vi "Axis_Jump Point.vi"(10 "Offset":T1, 11 "RobotPoints in":string[](array[string])) -> (0 "error out":errorcluster)   [LabVIEW 2019]
uses:
  LLB/Commonly VI/FilterPointNameToFloat.vi
panel:
  in  "error in (no error)":errorcluster
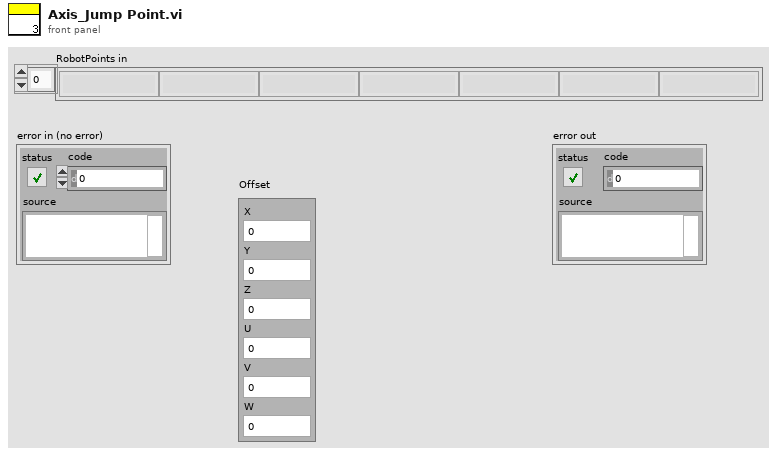
[diagram p1: front panel]
types:
  T1 = cluster{"X":dbl, "Y":dbl, "Z":dbl, "U":dbl, "V":dbl, "W":dbl}
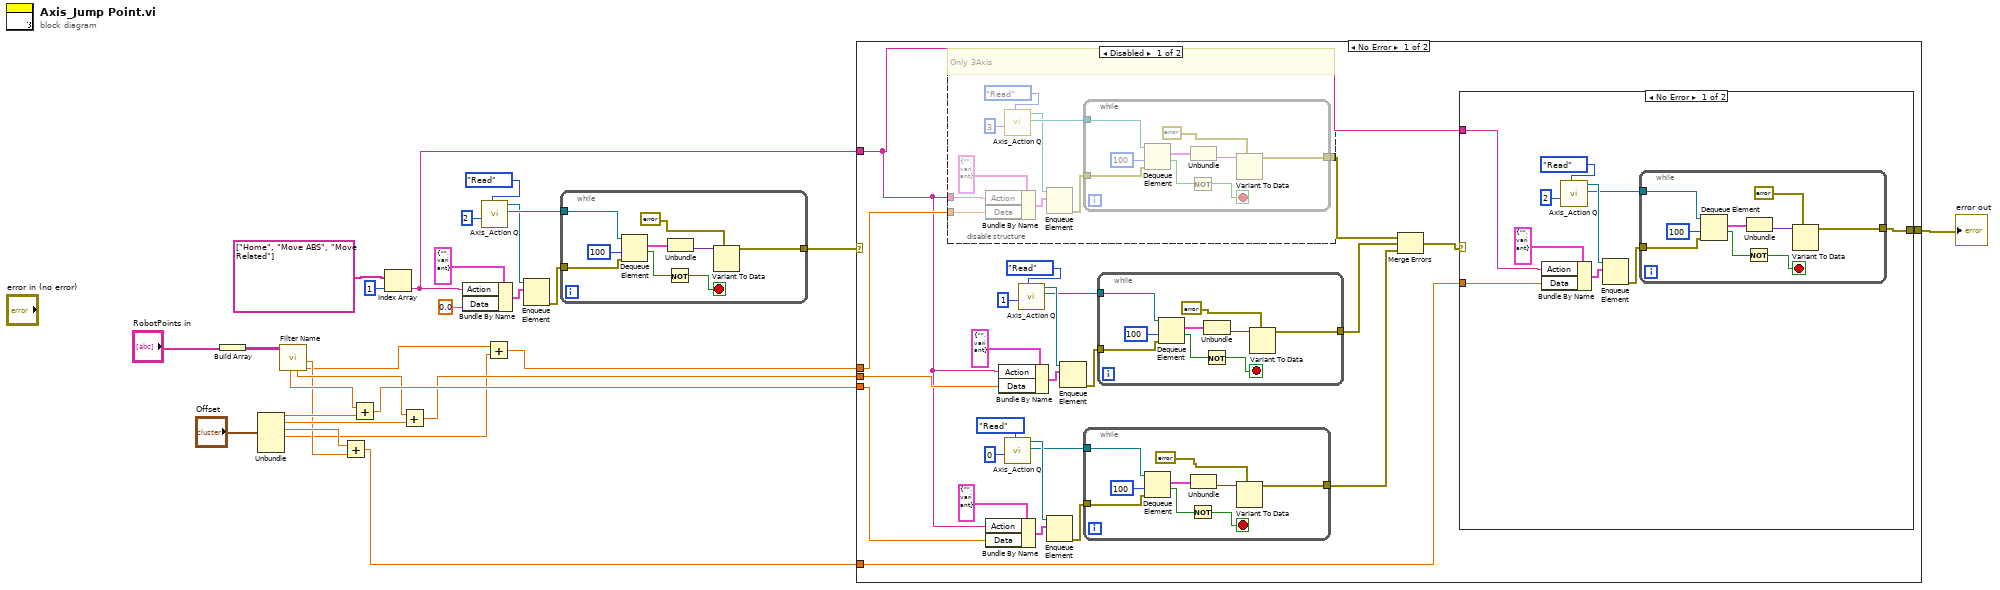
[diagram p0: block diagram]
diagram:
  n1 = Build Array("RobotPoints in") -> (w17:string[][])
  n2 = Unbundle("Offset") -> ("X"=w13:dbl, "Y"=w10:dbl, "Z"=w7:dbl, "U"=w3:dbl)  [unwired: 2 out]
  n3 = call-poly "Filter Name.vi"("RobotPoints in"=w17) -> ("U"=w2:dbl, "Z"=w6:dbl, "Y"=w9:dbl, "X"=w12:dbl)  [unwired: 4 in, 3 out]
  n4 = Add(x=w7, y=w6) -> (x+y=w5:dbl)
  n5 = Add(x=w12, y=w13) -> (x+y=w11:dbl)
  n6 = Index Array(array=string[] ["Home", "Move ABS", "Move Related"], index=1) -> (element=w18:string)
  n7 = Add(x=w9, y=w10) -> (x+y=w8:dbl)
  n8 = Bundle By Name(cluster=cluster{"Action":string, "Data":variant} {"Action"="", "Data"=variant} ("element"), "Action"=w18, "Data"=0.0) -> (w26:cluster{"Action":string, "Data":variant})
  n9 = call "Axis_Action Q.vi"("Enum"=enum16{"Initial", "Write", "Read"}."Read", "Axis Index"=2) -> ("Axis ActFeedBackQ Out"=w27:refnum<queue>, "Axis ActQ Out"=w25:refnum<queue>)  [unwired: 7 in, 1 out]
  n10 = Add(x=w2, y=w3) -> (x+y=w4:dbl)
  n11 = Enqueue Element(queue=w25, element=w26) -> (error out=w28:errorcluster)  [unwired: 2 in, 2 out]
  n12 = while {
    tunnel: w27 -> [w37]
    tunnel: w28 -> [w36]
    tunnel: [w29] -> w19
    stop <- w32 stop-if-true
    n13 = Dequeue Element(queue=w37, timeout in ms (-1)=100, error in (no error)=w36) -> (element=w34:cluster{"Action":string, "Data":variant}, timed out?=w33:bool)  [unwired: 2 out]
    n14 = Not(x=w33) -> (.not. x?=w32:bool)
    n15 = Unbundle(w34) -> ("Data"=w31:variant)  [unwired: 1 out]
    n16 = Variant To Data(type=errorcluster {"status"=FALSE, "code"=0, "source"=""} ("error constant"), Variant=w31) -> (data=w29:errorcluster)  [unwired: 1 in, 1 out]
  }
  n17 = case shown="No Error" w19 {
    selector: w19 -> [_ w119]
    tunnel: w18 -> [w40 _]
    tunnel: w11 -> [w47 _]
    tunnel: w8 -> [w46 _]
    tunnel: w4 -> [w45 _]
    tunnel: w5 -> [w39 _]
    tunnel: [w38 w119] -> w15
    frame No Error {
      n18 = disable-structure shown="Disabled" {
        disable-tunnel: w45 -> [w64 _]
        disable-tunnel: [w63 _] -> w44
        disable-tunnel: w40 -> [w62 _]
        frame Disabled {
          # "Only 3Axis"
          n19 = Bundle By Name(cluster=cluster{"Action":string, "Data":variant} {"Action"="", "Data"=variant} ("element"), "Action"=w62, "Data"=w64) -> (w69:cluster{"Action":string, "Data":variant})
          n20 = call "Axis_Action Q.vi"("Enum"=enum16{"Initial", "Write", "Read"}."Read", "Axis Index"=3) -> ("Axis ActFeedBackQ Out"=w70:refnum<queue>, "Axis ActQ Out"=w68:refnum<queue>)  [unwired: 7 in, 1 out]
          n21 = Enqueue Element(queue=w68, element=w69) -> (error out=w71:errorcluster)  [unwired: 2 in, 2 out]
          n22 = while {
            tunnel: w70 -> [w80]
            tunnel: w71 -> [w79]
            tunnel: [w72] -> w63
            stop <- w75 stop-if-true
            n23 = Dequeue Element(queue=w80, timeout in ms (-1)=100, error in (no error)=w79) -> (element=w77:cluster{"Action":string, "Data":variant}, timed out?=w76:bool)  [unwired: 2 out]
            n24 = Not(x=w76) -> (.not. x?=w75:bool)
            n25 = Unbundle(w77) -> ("Data"=w74:variant)  [unwired: 1 out]
            n26 = Variant To Data(type=errorcluster {"status"=FALSE, "code"=0, "source"=""} ("error constant"), Variant=w74) -> (data=w72:errorcluster)  [unwired: 1 in, 1 out]
          }
        }
        frame Enabled {
        }
      }
      n27 = Bundle By Name(cluster=cluster{"Action":string, "Data":variant} {"Action"="", "Data"=variant} ("element"), "Action"=w40, "Data"=w47) -> (w51:cluster{"Action":string, "Data":variant})
      n28 = Bundle By Name(cluster=cluster{"Action":string, "Data":variant} {"Action"="", "Data"=variant} ("element"), "Action"=w40, "Data"=w46) -> (w60:cluster{"Action":string, "Data":variant})
      n29 = call "Axis_Action Q.vi"("Enum"=enum16{"Initial", "Write", "Read"}."Read", "Axis Index"=0) -> ("Axis ActFeedBackQ Out"=w50:refnum<queue>, "Axis ActQ Out"=w53:refnum<queue>)  [unwired: 7 in, 1 out]
      n30 = call "Axis_Action Q.vi"("Enum"=enum16{"Initial", "Write", "Read"}."Read", "Axis Index"=1) -> ("Axis ActFeedBackQ Out"=w59:refnum<queue>, "Axis ActQ Out"=w61:refnum<queue>)  [unwired: 7 in, 1 out]
      n31 = Enqueue Element(queue=w53, element=w51) -> (error out=w49:errorcluster)  [unwired: 2 in, 2 out]
      n32 = Enqueue Element(queue=w61, element=w60) -> (error out=w58:errorcluster)  [unwired: 2 in, 2 out]
      n33 = while {
        tunnel: w50 -> [w109]
        tunnel: w49 -> [w108]
        tunnel: [w101] -> w42
        stop <- w104 stop-if-true
        n34 = Dequeue Element(queue=w109, timeout in ms (-1)=100, error in (no error)=w108) -> (element=w106:cluster{"Action":string, "Data":variant}, timed out?=w105:bool)  [unwired: 2 out]
        n35 = Not(x=w105) -> (.not. x?=w104:bool)
        n36 = Unbundle(w106) -> ("Data"=w103:variant)  [unwired: 1 out]
        n37 = Variant To Data(type=errorcluster {"status"=FALSE, "code"=0, "source"=""} ("error constant"), Variant=w103) -> (data=w101:errorcluster)  [unwired: 1 in, 1 out]
      }
      n38 = while {
        tunnel: w59 -> [w118]
        tunnel: w58 -> [w117]
        tunnel: [w110] -> w43
        stop <- w113 stop-if-true
        n39 = Dequeue Element(queue=w118, timeout in ms (-1)=100, error in (no error)=w117) -> (element=w115:cluster{"Action":string, "Data":variant}, timed out?=w114:bool)  [unwired: 2 out]
        n40 = Not(x=w114) -> (.not. x?=w113:bool)
        n41 = Unbundle(w115) -> ("Data"=w112:variant)  [unwired: 1 out]
        n42 = Variant To Data(type=errorcluster {"status"=FALSE, "code"=0, "source"=""} ("error constant"), Variant=w112) -> (data=w110:errorcluster)  [unwired: 1 in, 1 out]
      }
      n43 = Merge Errors(w44, w43, w42) -> (w41:errorcluster)
      n44 = case shown="No Error" w41 {
        selector: w41 -> [_ w100]
        tunnel: w40 -> [w83 _]
        tunnel: w39 -> [w82 _]
        tunnel: [w81 w100] -> w38
        frame No Error {
          n45 = Bundle By Name(cluster=cluster{"Action":string, "Data":variant} {"Action"="", "Data"=variant} ("element"), "Action"=w83, "Data"=w82) -> (w86:cluster{"Action":string, "Data":variant})
          n46 = call "Axis_Action Q.vi"("Enum"=enum16{"Initial", "Write", "Read"}."Read", "Axis Index"=2) -> ("Axis ActFeedBackQ Out"=w85:refnum<queue>, "Axis ActQ Out"=w87:refnum<queue>)  [unwired: 7 in, 1 out]
          n47 = Enqueue Element(queue=w87, element=w86) -> (error out=w84:errorcluster)  [unwired: 2 in, 2 out]
          n48 = while {
            tunnel: w85 -> [w99]
            tunnel: w84 -> [w98]
            tunnel: [w91] -> w81
            stop <- w94 stop-if-true
            n49 = Dequeue Element(queue=w99, timeout in ms (-1)=100, error in (no error)=w98) -> (element=w96:cluster{"Action":string, "Data":variant}, timed out?=w95:bool)  [unwired: 2 out]
            n50 = Not(x=w95) -> (.not. x?=w94:bool)
            n51 = Unbundle(w96) -> ("Data"=w93:variant)  [unwired: 1 out]
            n52 = Variant To Data(type=errorcluster {"status"=FALSE, "code"=0, "source"=""} ("error constant"), Variant=w93) -> (data=w91:errorcluster)  [unwired: 1 in, 1 out]
          }
        }
        frame Error {
        }
      }
    }
    frame Error {
    }
  }
  "error out" <- w15
